vi "Self_spi.vi"() -> ()   [LabVIEW 2015]
uses:
  <vilib>/Instr/_visa.llb/VISA Configure Serial Port (Instr).vi
  <vilib>/Utility/file.llb/Read Delimited Spreadsheet (I64).vi
panel:
  in  "write/read":enum16{"WRITE", "READ"}(ring)
  out "error_array":dbl[](array[numeric])
  in  "total":dbl
  in  "error":dbl
  out "VISA resource name out":refnum<visa-resource-name>
  in  "VISA resource name":refnum<visa-resource-name>="COM3"
  in  "save":bool
  in  "stop 3":bool
  out "data":string
  out "REG_V_U32":u32[](array[numeric])
  in  "stop 2":bool
  out "time":string
  in  "Write_data":string="0xff"
  in  "Reg Address":string="0x0000"
  in  "Block Address":string="0x08"
  in  "stop":bool
  in  "单次":bool
  out "R/W":i64[](array[numeric])
  out "REG_V_S":string[](array[string])
  out "r_com":string[](array[string])
  out "w_com":string[](array[string])
  out "num_of_reg":i32
  in  "测试写入数据":enum16{"0x55", "0xAA", "0xFF", "0x00"}(ring)
  out "Terminal Log 2":string="*IDN?"
  in  "Cycle Num":dbl(slide)=1.0 step=1.0 scale=0.0..20.0
  in  "DELAY(ms)":dbl(slide)=1.6161616161616161 scale=0.0..20.0 scale format="%#_4g"
  in  "寄存器连续读写测试报告路径":path=path "C:/Users/pigandhome/Desktop/Log.txt"
  in  "循环":bool
  out "all rows":i64[][](array[numeric])
  in  "寄存器List":path=path "C:/Users/pigandhome/Desktop/Everst_REG_ALL.xls"
  in  "停止":bool
  out "Terminal1":string="*IDN?"
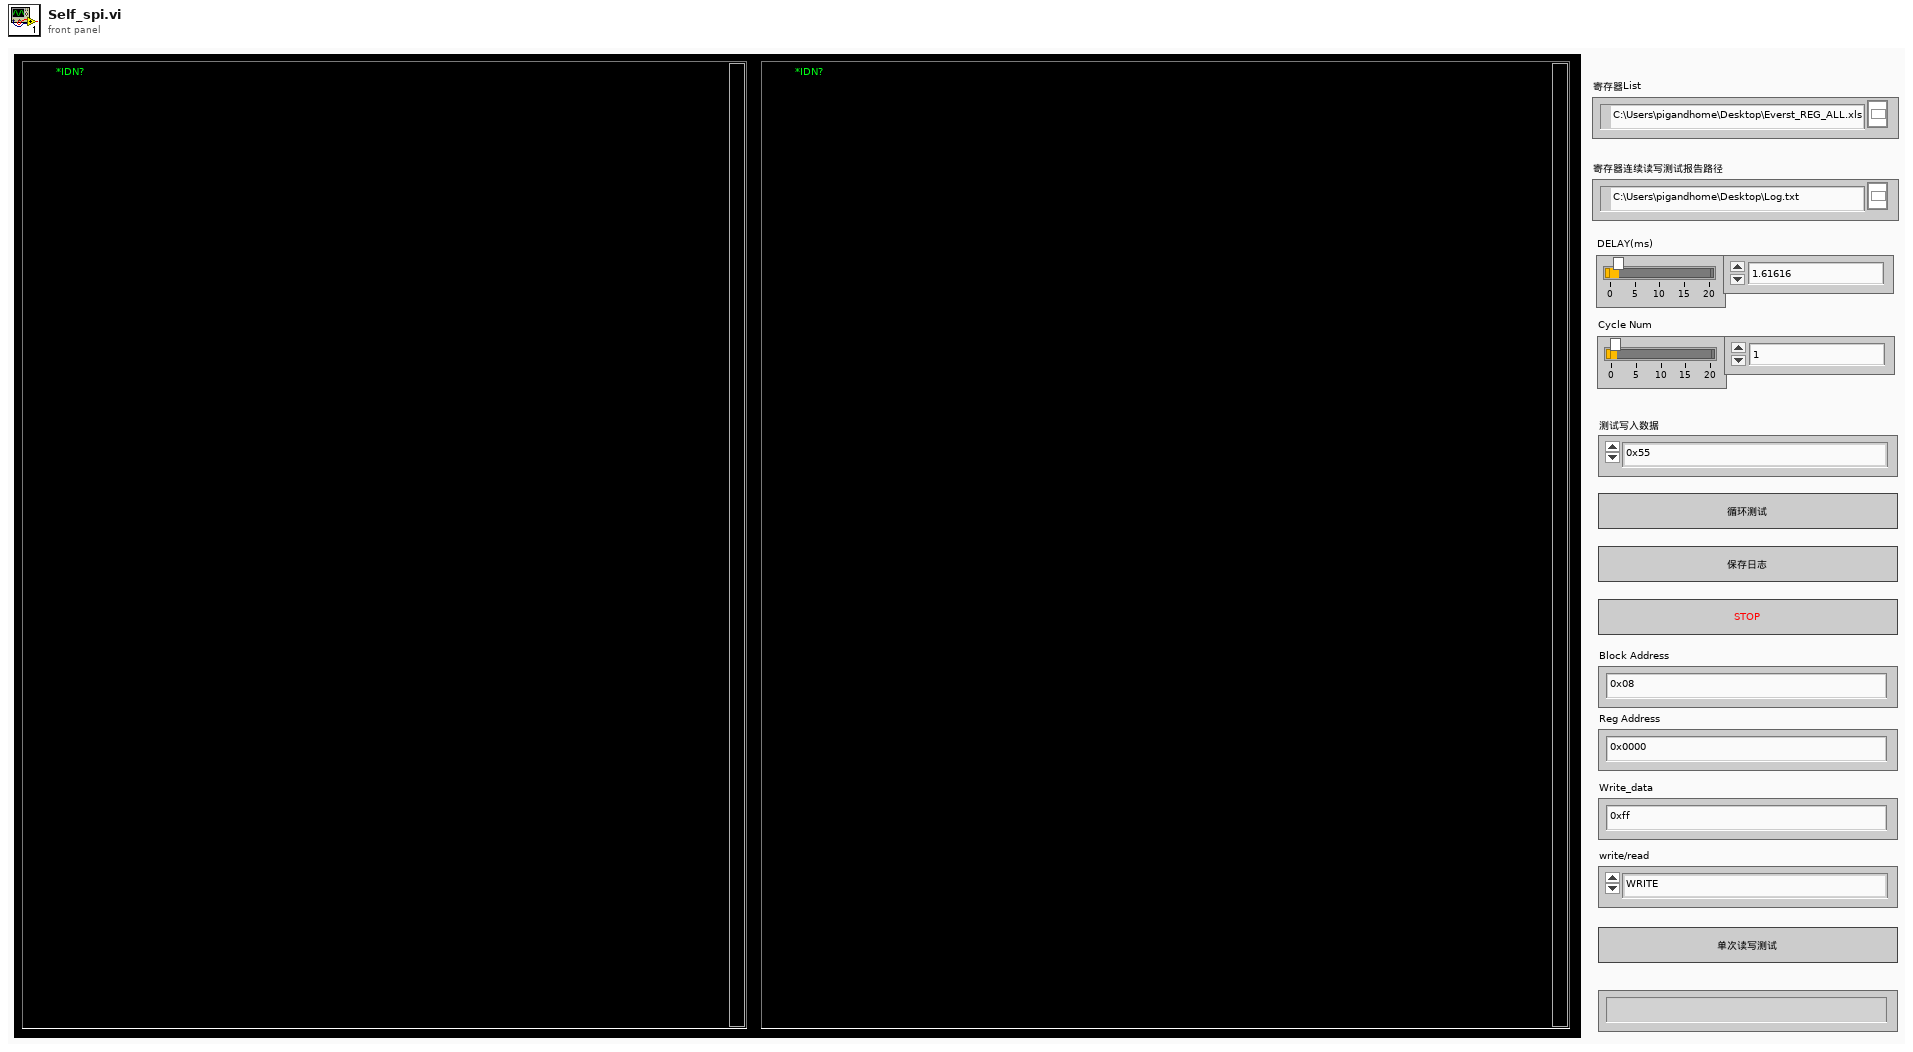
[diagram p1: front panel]
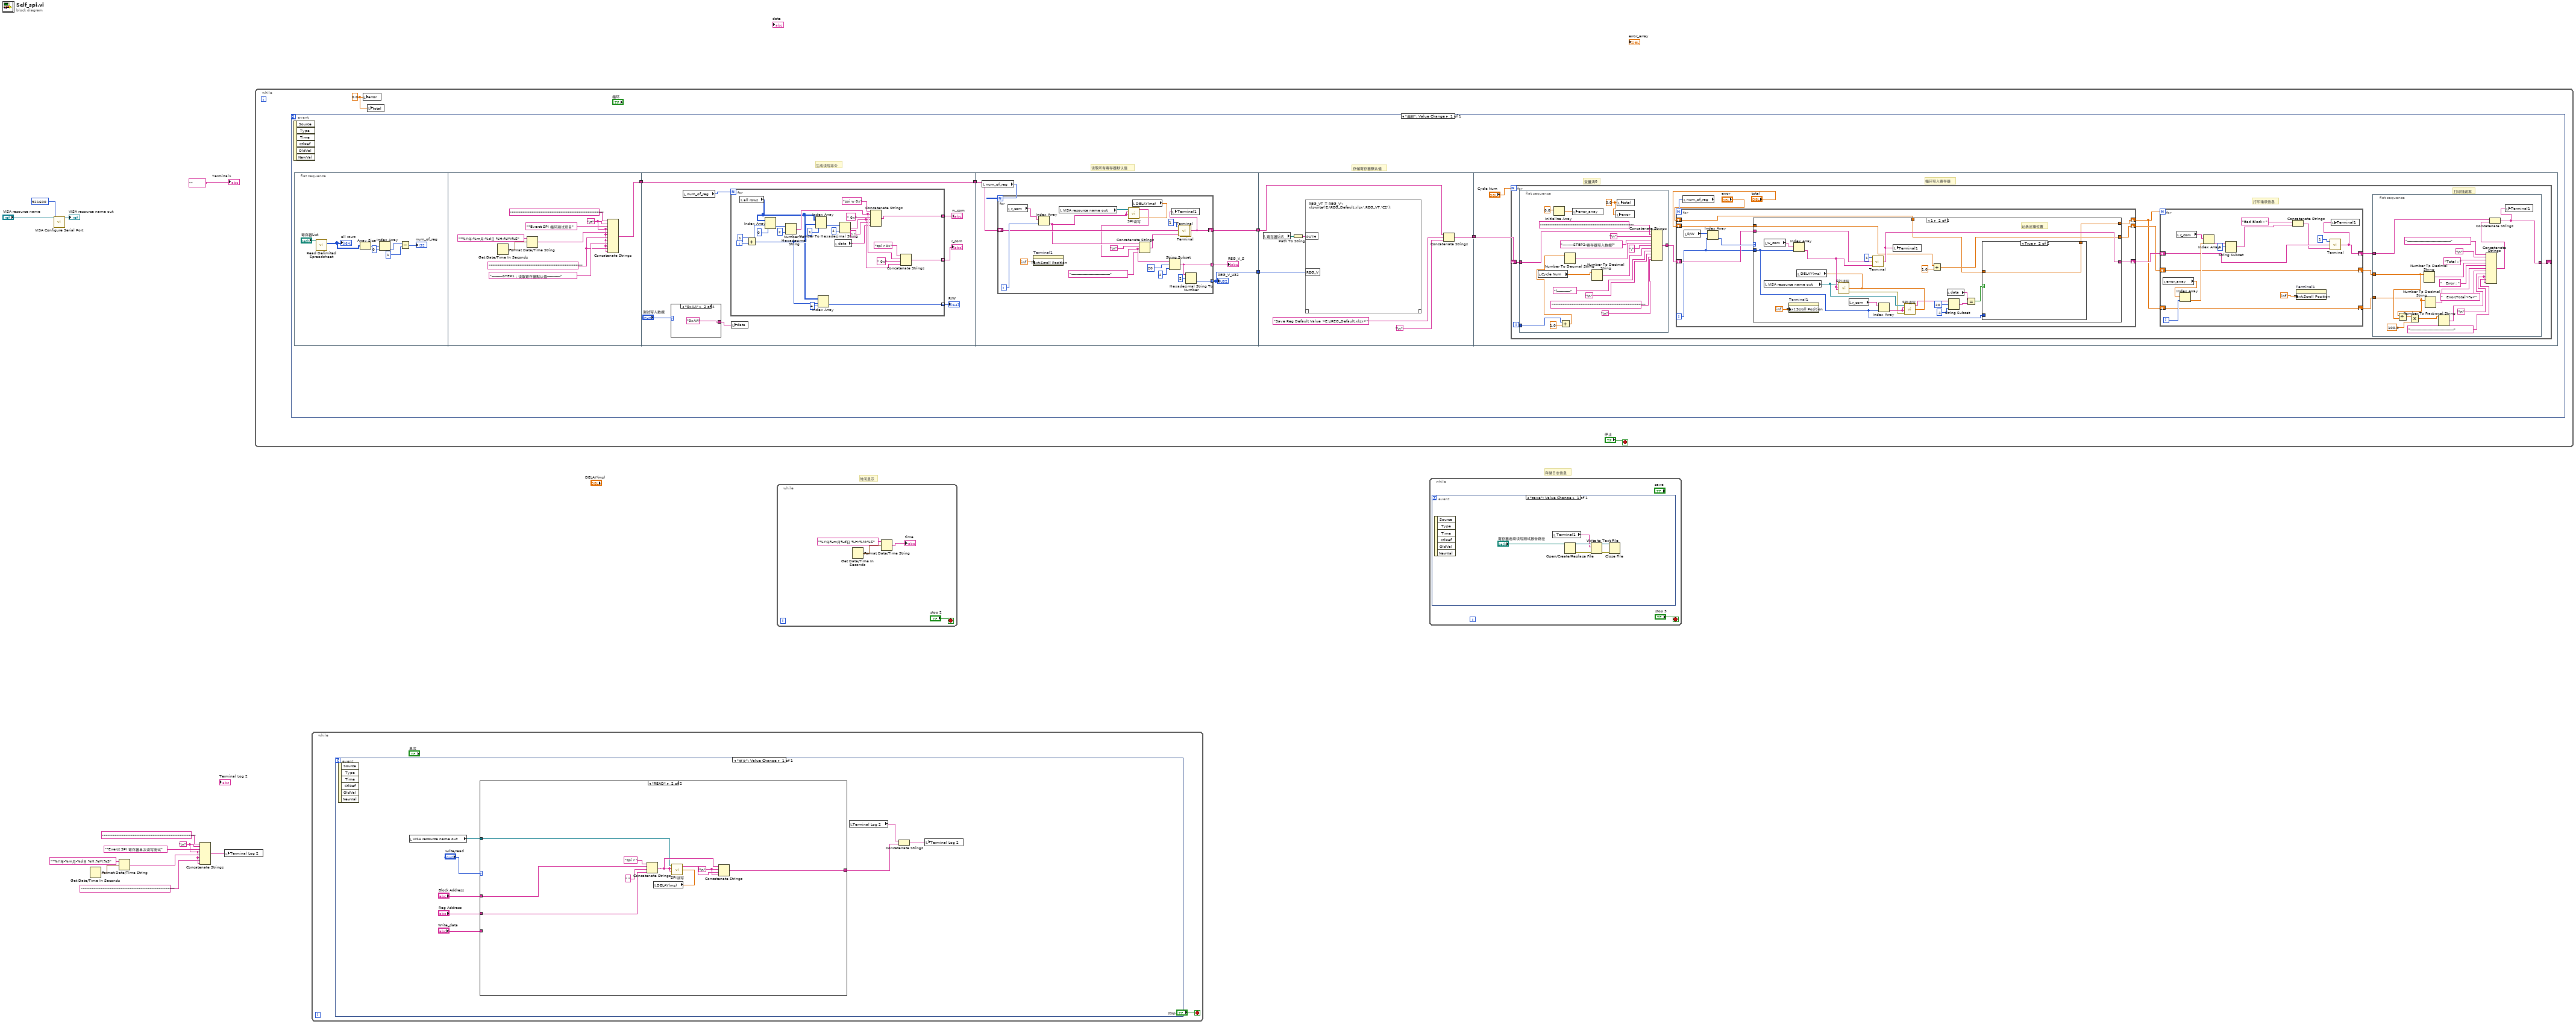
[diagram p0: block diagram]
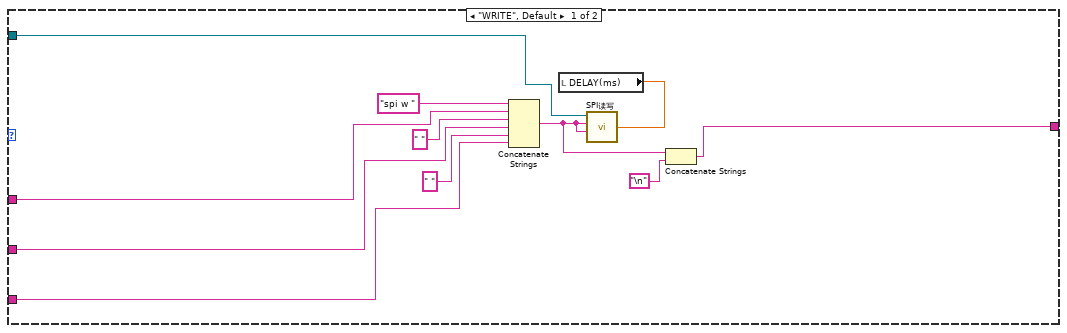
[diagram p2: hidden frame]
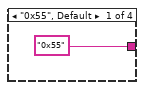
[diagram p3: hidden frame]
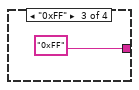
[diagram p4: hidden frame]
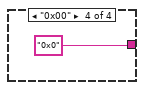
[diagram p5: hidden frame]
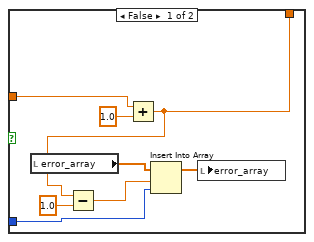
[diagram p7: hidden frame]
diagram:
  w6 = "\n"
  # "时间显示"
  # "存储日志信息"
  n1 = call-poly "VISA Configure Serial Port"("VISA resource name"="VISA resource name", "baud rate (9600)"=u32 921600) -> ("VISA resource name out"=→"VISA resource name out":refnum<visa-resource-name>)  [unwired: 12 in, 1 out]
  n2 = Get Date/Time In Seconds() -> (seconds since 1Jan1904=w10:timestamp)
  n3 = Format Date/Time String(time format string (%c)="*%Y年-%m月-%d日 %H:%M:%S", seconds (now)=w10) -> (date/time string=w8:string)  [unwired: 1 in]
  n4 = Concatenate Strings("**************************************************" ("string"), w6, "*Everst SPI 寄存器单次读写测试" ("string"), w6, w8, w6, "**************************************************" ("string"), w6) -> (w5:string)
  n5 = local write "Terminal Log 2"(w5) -> ()
  n6 = while {
    stop <- "停止" stop-if-true
    w13 = 0.0 ("error")
    n7 = event shown="[0] \"循环\": Value Change" {
      selector: _ -> [_]
      dyn-events: _ -> [_]
      timeout: _ -> [_]
      event "循环": Value Change {
        # "存储寄存器默认值"
        # "读取所有寄存器默认值"
        # "生成读写命令"
        n8 = event-data() -> ()  [unwired: 1 in, 6 out]
        n9 = flat-sequence {
          tunnel: [w30] -> w18
          tunnel: [w39] -> w19
          tunnel: w18 -> [w39]
          tunnel: w19 -> [w73]
          tunnel: [w70] -> w17
          tunnel: [w69] -> w15
          tunnel: w17 -> [w98]
          tunnel: [w93] -> w16
          tunnel: w15 -> [w95]
          tunnel: w16 -> [w99]
          frame #0 {
            n10 = call-poly <vilib>:"Read Delimited Spreadsheet.vi"("file path (dialog if empty)"="寄存器List") -> ("all rows"=w21:i64[][])  [unwired: 9 in, 5 out]
            "all rows" <- w21
            n11 = Array Size(array=w21) -> (size(s)=w23:i32[])
            n12 = Index Array(array=w23, index=0) -> (element=w24:i32)
            n13 = Subtract(x=w24, y=1) -> (x-y=→"num_of_reg":i32)
          }
          frame #1 {
            w28 = "**************************************************" ("string")
            w27 = "\n"
            n14 = Get Date/Time In Seconds() -> (seconds since 1Jan1904=w33:timestamp)
            n15 = Format Date/Time String(time format string (%c)="*%Y年-%m月-%d日 %H:%M:%S", seconds (now)=w33) -> (date/time string=w35:string)  [unwired: 1 in]
            n16 = Concatenate Strings("**************************************************" ("string"), w27, "*Everst SPI 循环测试项目" ("string"), w27, w35, w27, w28, w27, "---------STEP1：读取寄存器默认值-----------" ("string"), w27, w28, w27) -> (w30:string)
          }
          frame #2 {
            n17 = case shown="\"0xAA\"" "测试写入数据" {
              tunnel: ["0x55" "0xAA" "0xFF" "0x0"] -> w36
              frame "0x55", Default {
              }
              frame "0xAA" {
              }
              frame "0xFF" {
              }
              frame "0x00" {
              }
            }
            n18 = local read "num_of_reg"() -> (w38:i32)
            n19 = for {
              N: w38 -> [_]
              tunnel: [w54] -> w42 mode=indexing
              tunnel: [w53] -> w41 mode=indexing
              tunnel: [w48] -> w40 mode=indexing
              i -> [w60]
              n20 = local read "all rows"() -> (w50:i64[][])
              n21 = Add(x=1, y=w60) -> (x+y=w51:i32)
              n22 = Index Array(array=w50, index (row)=w51, index (col)=0 ("disabled index (col)")) -> (element=w67:i64)
              n23 = Number To Hexadecimal String(1:i16 2 ("width (-)"), 2:w67) -> (0:w56:string)
              n24 = Index Array(array=w50, index (row)=w51, index (col)=1 ("disabled index (col)")) -> (element=w63:i64)
              n25 = Index Array(array=w50, index (row)=w51, index (col)=4 ("disabled index (col)")) -> (element=w48:i64)
              n26 = local read "data"() -> (w47:string)
              n27 = Number To Hexadecimal String(1:i16 4 ("width (-)"), 2:w63) -> (0:w52:string)
              n28 = Concatenate Strings("spi w 0x" ("string"), w56, " 0x" ("string"), w52, " " ("string"), w47) -> (w54:string)
              n29 = Concatenate Strings("spi r 0x" ("string"), w56, " 0x" ("string"), w52) -> (w53:string)
            }
            "w_com" <- w42
            "r_com" <- w41
            "R/W" <- w40
            n30 = local write "data"(w36) -> ()
          }
          frame #3 {
            n31 = local read "num_of_reg"() -> (w72:i32)
            n32 = for {
              N: w72 -> [_]
              shift-right: [w88] -> w69
              shift-left: w73 -> [w90]
              tunnel: [w82] -> w71 mode=indexing
              tunnel: [w80] -> w70 mode=indexing
              i -> [w91]
              n33 = local read "r_com"() -> (w87:string[])
              n34 = property on="Terminal1" class="Str"("Text.Scroll Position"=inf) -> ()  [unwired: 2 in, 2 out]
              n35 = Index Array(array=w87, index=w91) -> (element=w78:string)
              n36 = local read "VISA resource name out"() -> (w79:refnum<visa-resource-name>)
              n37 = local read "DELAY(ms)"() -> (w75:dbl)
              n38 = call "SPI读写.vi"("DELAY"=w75, "从芯片读数据"=w78, "往芯片写数据"=w78, "VISA resource name"=w79) -> ("read buffer"=w77:string)  [unwired: 1 in, 1 out]
              n39 = Concatenate Strings(w78, "\n", w77, "--------------------------------" ("string")) -> (w86:string)
              n40 = String Subset(string=w77, offset (0)=20, length (rest)=4 ("length (rest)")) -> (substring=w82:string)
              n41 = call "Terminal.vi"("Add"=w86, "Head"=w90, "LINE"=1) -> ("Str Out"=w88:string)
              n42 = local write "Terminal1"(w88) -> ()
              n43 = call "Terminal.vi"() -> ()  [unwired: 3 in, 1 out]
              n44 = Hexadecimal String To Number(string=w82, offset=2) -> (number=w80:u32)  [unwired: 1 in, 1 out]
            }
            "REG_V_S" <- w71
            "REG_V_U32" <- w70
          }
          frame #4 {
            n45 = local read "寄存器List"() -> (w96:path)
            n46 = Path To String(path=w96) -> (string=w97:string)
            n47 = script code="REG_VT = REG_V';\nxlswrite('E:\\REG_Default.xlsx',REG_VT,'C2');"("REG_V"=w98, "PATH"=w97) -> ()  [unwired: 1 in, 1 out]
            n48 = Concatenate Strings(w95, "Save Reg Default Value <E:\\REG_Default.xlsx>" ("string"), "\n") -> (w93:string)
          }
          frame #5 {
            # "变量清0"
            # "循环写入寄存器"
            n49 = for {
              N: "Cycle Num" -> [_]
              shift-right: [w108] -> _
              shift-left: w99 -> [w112]
              i -> [w111]
              # "打印错误率"
              # "打印错误信息"
              n50 = flat-sequence {
                tunnel: [w188] -> w113
                tunnel: w112 -> [w183]
                tunnel: w111 -> [w180]
                frame #0 {
                  w177 = 0.0 ("total")
                  n51 = local read "Cycle Num"() -> (w181:dbl)
                  n52 = Initialize Array(0.0 ("element")) -> (w176:dbl[])  [unwired: 1 in]
                  n53 = Add(x=w180, y=1.0) -> (x+y=w179:dbl)
                  n54 = Number To Decimal String(number=w179) -> (decimal integer string=w193:string)  [unwired: 1 in]
                  n55 = local write "error_array"(w176) -> ()
                  n56 = Number To Decimal String(number=w181) -> (decimal integer string=w191:string)  [unwired: 1 in]
                  n57 = local write "error"(w177) -> ()
                  n58 = local write "total"(w177) -> ()
                  n59 = Concatenate Strings(w183, "**************************************************" ("string"), "\n", "---------STEP2:寄存器写入数据(" ("string"), w193, "/" ("string"), w191, ")-----------" ("string"), "\n", "**************************************************" ("string"), "\n") -> (w188:string)
                }
              }
              n60 = local read "num_of_reg"() -> (w107:i32)
              n61 = for {
                N: w107 -> [_]
                shift-right: [w119] -> w110
                shift-left: w113 -> [w120]
                shift-right: [w114] -> w101
                shift-left: "error" -> [w115]
                shift-right: [w116] -> w104
                shift-left: "total" -> [w117]
                i -> [w118]
                n62 = local read "R/W"() -> (w122:i64[])
                n63 = Index Array(array=w122, index=w118) -> (element=w121:i64)
                n64 = case shown="1" w121 {
                  tunnel: w118 -> [_ w131]
                  tunnel: w120 -> [w125 w147]
                  tunnel: [w125 w133] -> w119
                  tunnel: w117 -> [w124 w129]
                  tunnel: [w124 w128] -> w116
                  tunnel: w115 -> [w123 w127]
                  tunnel: [w123 w126] -> w114
                  frame 0, Default {
                  }
                  frame 1 {
                    # "记录出错位置"
                    n65 = local read "w_com"() -> (w148:string[])
                    n66 = local read "VISA resource name out"() -> (w141:refnum<visa-resource-name>)
                    n67 = property on="Terminal1" class="Str"("Text.Scroll Position"=inf) -> ()  [unwired: 2 in, 2 out]
                    n68 = Index Array(array=w148, index=w131) -> (element=w145:string)
                    n69 = local read "DELAY(ms)"() -> (w140:dbl)
                    n70 = call "SPI读写.vi"("DELAY"=w140, "从芯片读数据"=w145, "往芯片写数据"=w145, "VISA resource name"=w141) -> ("error out"=w130:errorcluster)  [unwired: 1 in, 1 out]
                    n71 = local read "r_com"() -> (w143:string[])
                    n72 = call "Terminal.vi"("Add"=w145, "Head"=w147, "LINE"=1) -> ("Str Out"=w133:string)
                    n73 = Index Array(array=w143, index=w131) -> (element=w142:string)
                    n74 = local write "Terminal1"(w133) -> ()
                    n75 = call "SPI读写.vi"("DELAY"=w140, "error in (no error)"=w130, "从芯片读数据"=w142, "往芯片写数据"=w142, "VISA resource name"=w141) -> ("read buffer"=w139:string)  [unwired: 1 out]
                    n76 = Add(x=w129, y=1.0) -> (x+y=w128:dbl)
                    n77 = local read "data"() -> (w135:string)
                    n78 = String Subset(string=w139, offset (0)=20, length (rest)=4 ("length (rest)")) -> (substring=w136:string)
                    n79 = Equal?(x=w135, y=w136) -> (x = y?=w134:bool)
                    n80 = case shown="True" w134 {
                      tunnel: w131 -> [w152 _]
                      tunnel: w127 -> [w150 w157]
                      tunnel: [w149 w157] -> w126
                      frame False {
                        n81 = local read "error_array"() -> (w151:dbl[])
                        n82 = Add(x=w150, y=1.0) -> (x+y=w149:dbl)
                        n83 = Subtract(x=w149, y=1.0) -> (x-y=w154:dbl)
                        n84 = Insert Into Array(array=w151, index=w154, new element=w152) -> (w153:dbl[])
                        n85 = local write "error_array"(w153) -> ()
                      }
                      frame True {
                      }
                    }
                  }
                }
              }
              n86 = for {
                N: w101 -> [_]
                shift-right: [w198] -> w109
                shift-left: w110 -> [w200]
                shift-right: [w197] -> w103
                shift-left: w104 -> [w197]
                shift-right: [w196] -> w102
                shift-left: w101 -> [w196]
                i -> [w208]
                n87 = local read "error_array"() -> (w207:dbl[])
                n88 = local read "r_com"() -> (w209:string[])
                n89 = Index Array(array=w207, index=w208) -> (element=w206:dbl)
                n90 = Index Array(array=w209, index=w206) -> (element=w204:string)
                n91 = String Subset(string=w204, offset (0)=6) -> (substring=w202:string)  [unwired: 1 in]
                n92 = Concatenate Strings("Bad Block : " ("string"), w202) -> (w199:string)
                n93 = property on="Terminal1" class="Str"("Text.Scroll Position"=inf) -> ()  [unwired: 2 in, 2 out]
                n94 = call "Terminal.vi"("Add"=w199, "Head"=w200, "LINE"=1) -> ("Str Out"=w198:string)
                n95 = local write "Terminal1"(w198) -> ()
              }
              n96 = flat-sequence {
                tunnel: w109 -> [w162]
                tunnel: [w161] -> w108
                tunnel: w103 -> [w160]
                tunnel: w102 -> [w159]
                frame #0 {
                  w166 = "\n"
                  n97 = Divide(x=w159, y=w160) -> (x/y=w165:dbl)
                  n98 = Multiply(x=w165, y=100.0) -> (x*y=w164:dbl)
                  n99 = Number To Decimal String(number=w160) -> (decimal integer string=w172:string)  [unwired: 1 in]
                  n100 = Number To Decimal String(number=w159) -> (decimal integer string=w170:string)  [unwired: 1 in]
                  n101 = Number To Fractional String(number=w164) -> (F-format string=w168:string)  [unwired: 3 in]
                  n102 = Concatenate Strings("------------------------------------" ("string"), "\n", "Total : " ("string"), w172, "   Error : " ("string"), w170, "   Error/Total<%>" ("string"), w168, w166, "------------------------------------" ("string"), w166) -> (w158:string)
                  n103 = Concatenate Strings(w162, w158) -> (w161:string)
                  n104 = local write "Terminal1"(w161) -> ()
                }
              }
            }
          }
        }
      }
    }
    n105 = local write "error"(w13) -> ()
    n106 = local write "total"(w13) -> ()
  }
  n107 = while {
    stop <- "stop" stop-if-true
    n108 = event shown="[0] \"单次\": Value Change" {
      selector: _ -> [_]
      dyn-events: _ -> [_]
      timeout: _ -> [_]
      event "单次": Value Change {
        n109 = event-data() -> ()  [unwired: 1 in, 6 out]
        n110 = local read "VISA resource name out"() -> (w211:refnum<visa-resource-name>)
        n111 = case shown="\"READ\"" "write/read" {
          tunnel: "Block Address" -> [w226 w237]
          tunnel: "Reg Address" -> [w225 w236]
          tunnel: [w221 w232] -> w215
          tunnel: "Write_data" -> [w224 _]
          tunnel: w211 -> [w219 w230]
          frame "WRITE", Default {
            n112 = Concatenate Strings("spi w " ("string"), w226, " " ("string"), w225, " " ("string"), w224) -> (w222:string)
            n113 = local read "DELAY(ms)"() -> (w220:dbl)
            n114 = call "SPI读写.vi"("DELAY"=w220, "从芯片读数据"=w222, "往芯片写数据"=w222, "VISA resource name"=w219) -> ()  [unwired: 1 in, 2 out]
            n115 = Concatenate Strings(w222, "\n") -> (w221:string)
          }
          frame "READ" {
            w233 = "\n"
            n116 = Concatenate Strings("spi r " ("string"), w237, " " ("string"), w236) -> (w235:string)
            n117 = local read "DELAY(ms)"() -> (w231:dbl)
            n118 = call "SPI读写.vi"("DELAY"=w231, "从芯片读数据"=w235, "往芯片写数据"=w235, "VISA resource name"=w230) -> ("read buffer"=w234:string)  [unwired: 1 in, 1 out]
            n119 = Concatenate Strings(w235, w233, w234, w233) -> (w232:string)
          }
        }
        n120 = local read "Terminal Log 2"() -> (w213:string)
        n121 = Concatenate Strings(w213, w215) -> (w214:string)
        n122 = local write "Terminal Log 2"(w214) -> ()
      }
    }
  }
  n123 = while {
    stop <- "stop 2" stop-if-true
    n124 = Get Date/Time In Seconds() -> (seconds since 1Jan1904=w242:timestamp)
    n125 = Format Date/Time String(time format string (%c)="%Y年%m月%d日 %H:%M:%S", seconds (now)=w242) -> (date/time string=→"time":string)  [unwired: 1 in]
  }
  n126 = while {
    stop <- "stop 3" stop-if-true
    n127 = event shown="[0] \"save\": Value Change" {
      selector: _ -> [_]
      dyn-events: _ -> [_]
      timeout: _ -> [_]
      event "save": Value Change {
        n128 = event-data() -> ()  [unwired: 1 in, 6 out]
        n129 = local read "Terminal1"() -> (w248:string)
        n130 = Open/Create/Replace File(file path (use dialog)="寄存器连续读写测试报告路径") -> (refnum out=w249:refnum<file>, error out=w250:errorcluster)  [unwired: 5 in, 1 out]
        n131 = Write to Text File(file (use dialog)=w249, text=w248, error in=w250) -> (refnum out=w246:refnum<file>, error out=w247:errorcluster)  [unwired: 1 in, 1 out]
        n132 = Close File(refnum=w246, error in=w247) -> ()  [unwired: 2 out]
      }
    }
  }
  "Terminal1" <- "" ("Terminal1")
